vi "Write create file if necessary.vi"(8 "error in (no error)":errorcluster, 10 "create file if necessary (T)":bool=TRUE, 11 "INIFileClass in":refnum<class "INIFileClass.lvclass">) -> (0 "error out":errorcluster, 3 "INIFileClass out":refnum<class "INIFileClass.lvclass">)   [LabVIEW 2013, in "INIFileClass.lvclass"]
uses:
  INIFileClass.lvclass
  INIFileClass.lvclass/INIFileClass.ctl
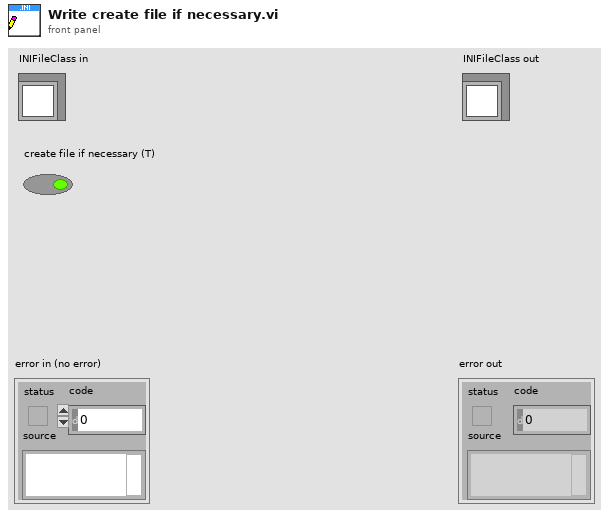
[diagram p1: front panel]
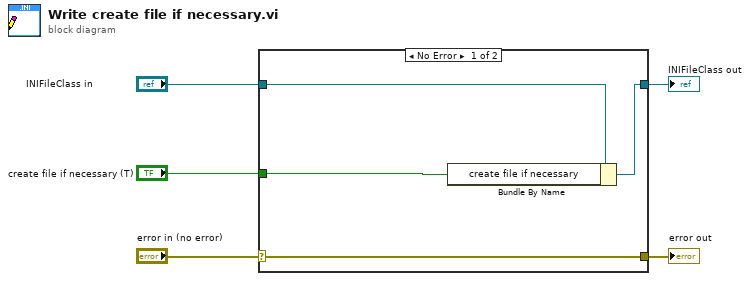
[diagram p0: block diagram]
diagram:
  n1 = case shown="No Error" "error in (no error)" {
    selector: "error in (no error)" -> [w9 w10]
    tunnel: [w9 w10] -> w4
    tunnel: [w7 w11] -> w2
    tunnel: "INIFileClass in" -> [w8 w11]
    tunnel: "create file if necessary (T)" -> [w6 _]
    frame No Error {
      n2 = Bundle By Name(cluster=w8, "create file if necessary"=w6) -> (w7:refnum<class "INIFileClass.lvclass">)
    }
    frame Error {
    }
  }
  "error out" <- w4
  "INIFileClass out" <- w2
